vi "Add Correction.vi"(8 "error in (no error)":errorcluster, 10 "XYZTheta":dbl[](array[numeric]), 11 "Carrier Tray in":refnum<class "Assembly Tray.lvclass">) -> (0 "error out":errorcluster, 2 "XYZTheta Out":dbl[](array[numeric]), 3 "Carrier Tray out":refnum<class "Assembly Tray.lvclass">)   [LabVIEW 2020, in "Assembly Tray.lvclass"]
uses:
  Assembly Tray.lvclass
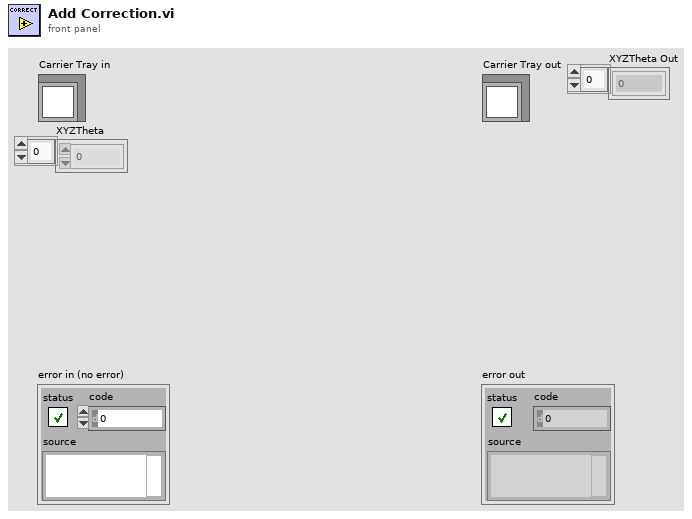
[diagram p1: front panel]
types:
  T1 = typedef "File Paths.ctl" = cluster{"Glue Pattern Folder":path, "Carrier Tray Folder":path, "Pick Up Tool Fixture Folder":path, "Components Folder":path, "Bellows Tool Offset.txt":path, "Pick Up Tool Offset.txt":path, "Dispense Tip Offset.txt":path, "Log Files":path, "Gantry Assembly Map.txt":path, "Syringe and offset map.txt":path}
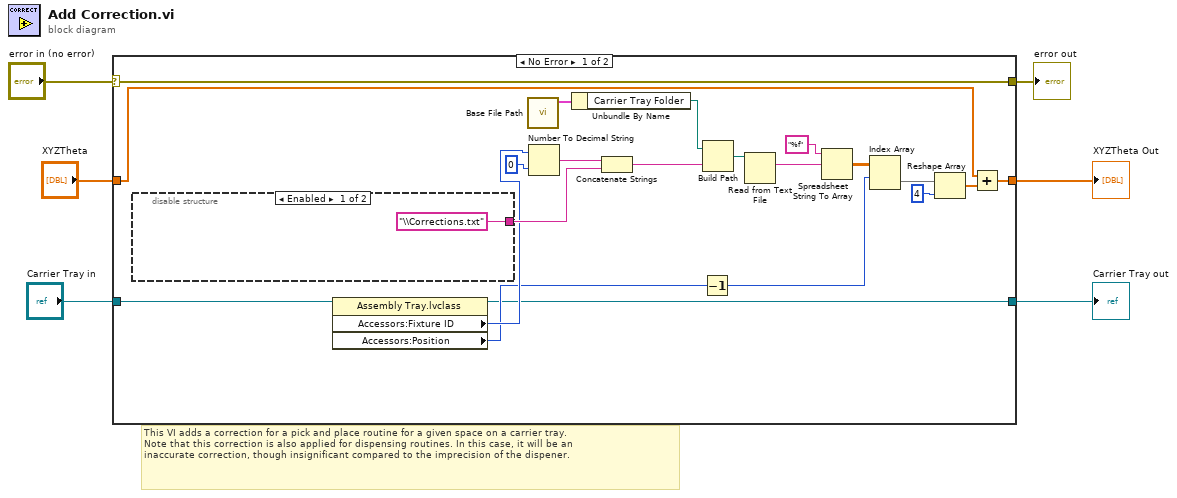
[diagram p0: block diagram]
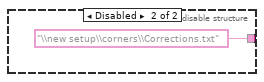
[diagram p2: hidden frame]
diagram:
  # "This VI adds a correction for a pick and place routine for a given space on a carrier tray.\nNote that this correction is also applied for dispensing routines. In this case, it will be an\ninaccurate correction, though insignificant compared to the imprecision of the dispener."
  n1 = case shown="No Error" "error in (no error)" {
    selector: "error in (no error)" -> [w27 w32]
    tunnel: [w27 w32] -> w5
    tunnel: [w7 w31] -> w3
    tunnel: "Carrier Tray in" -> [w10 w31]
    tunnel: "XYZTheta" -> [w13 w30]
    tunnel: [w11 w30] -> w1
    frame No Error {
      n2 = disable-structure shown="Enabled" {
        disable-tunnel: ["\\Corrections.txt" ("name or relative path") "\\new setup\\corners\\Corrections.txt" ("name or relative path")] -> w22
        frame Enabled {
        }
        frame Disabled {
        }
      }
      n3 = property class="Assembly Tray.lvclass"(reference=w10) -> (reference out=w7:refnum<class "Assembly Tray.lvclass">, "Accessors:Fixture ID"=w9:i32, "Accessors:Position"=w8:i32)  [unwired: 1 in, 1 out]
      n4 = call "Base File Path.vi"() -> ("Paths Out"=w26:T1)  [unwired: 11 in]
      n5 = Number To Decimal String(number=w9, width (-)=i16 0) -> (decimal integer string=w23:string)
      n6 = Unbundle By Name(w26) -> ("Carrier Tray Folder"=w25:path)
      n7 = Concatenate Strings(w23, w22) -> (w21:string)
      n8 = Decrement(x=w8) -> (x-1=w16:i32)
      n9 = Build Path(base path=w25, name or relative path=w21) -> (appended path=w20:path)
      n10 = Read from Text File(file (use dialog)=w20) -> (text=w19:string)  [unwired: 3 in, 3 out]
      n11 = Spreadsheet String To Array(format string="%f", spreadsheet string=w19) -> (array=w17:dbl[][])  [unwired: 2 in]
      n12 = Index Array(array=w17, index (row)=w16) -> (element=w14:dbl[])  [unwired: 1 in]
      n13 = Reshape Array(w14, 4 ("dimension size")) -> (w12:dbl[])
      n14 = Add(x=w13, y=w12) -> (x+y=w11:dbl[])
    }
    frame Error {
    }
  }
  "error out" <- w5
  "Carrier Tray out" <- w3
  "XYZTheta Out" <- w1
